vi "Demo.vi"() -> ()   [LabVIEW 2018]
doc: "Example API Tester."
uses:
  Classes/ExampleAPI/ExampleAPI.lvclass
panel:
  in  "Get Bitness Info":bool
  in  "machine name (\"\":  local reference)":string="localhost"
  in  "port number":u16=3365
  in  "wait for reply":bool=TRUE
  in  "X":dbl=1.0
  out "Reply Payload":dbl
  in  "Stop Module":bool
  in  "Test Do Something Else and Wait for Reply":bool
  in  "Hide Module Panel":bool
  in  "Show Module Panel":bool
  in  "Test Do Something Else":bool
  in  "Test Do Something":bool
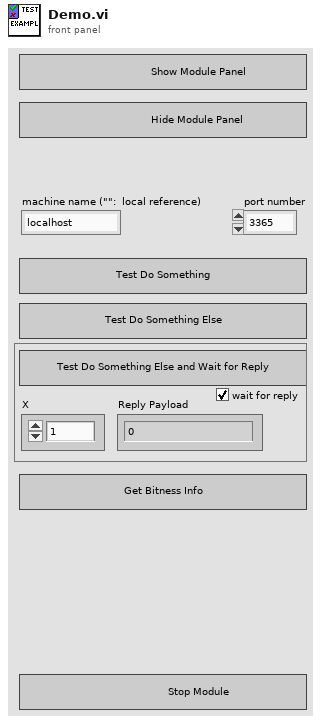
[diagram p1: front panel]
types:
  T1 = typedef "Example.lvlib/Do Something Else and Wait (Reply Payload)--cluster.ctl" = cluster{"Value":dbl, "error":errorcluster}
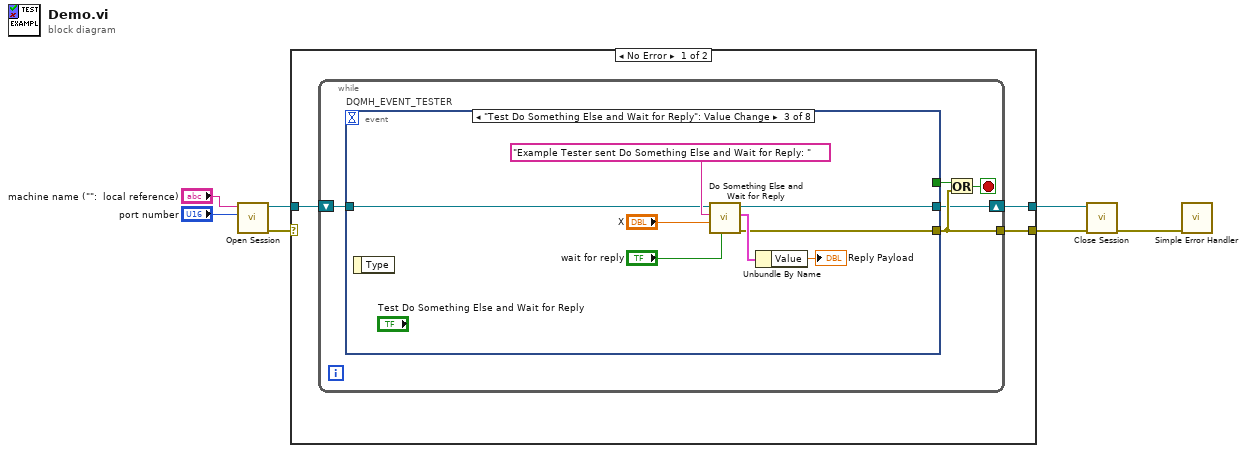
[diagram p0: block diagram]
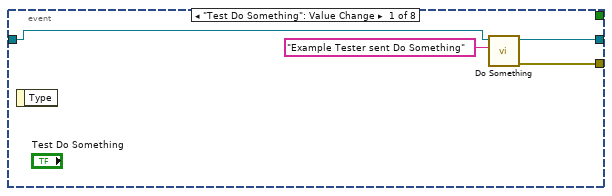
[diagram p2: hidden frame]
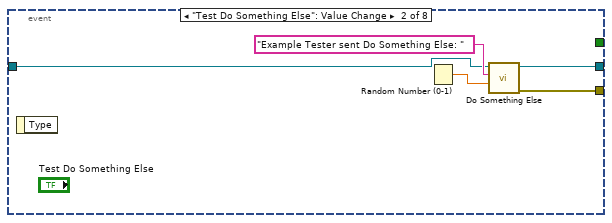
[diagram p3: hidden frame]
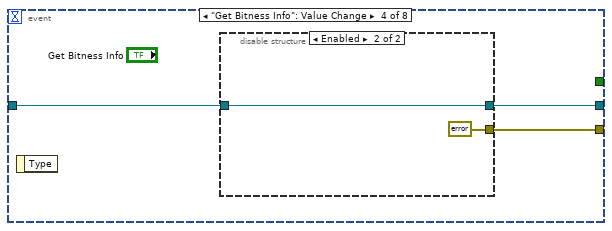
[diagram p4: hidden frame]
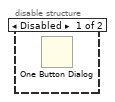
[diagram p5: hidden frame]
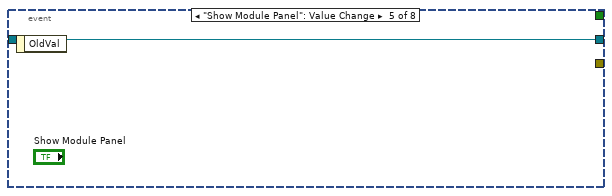
[diagram p6: hidden frame]
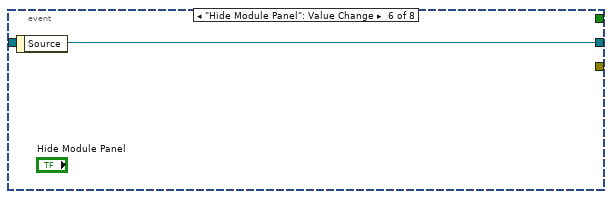
[diagram p7: hidden frame]
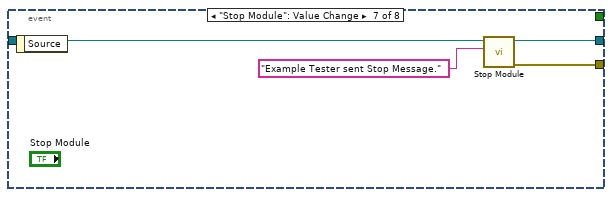
[diagram p8: hidden frame]
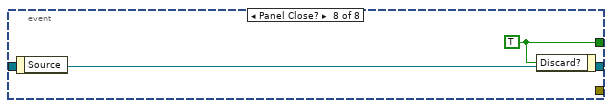
[diagram p9: hidden frame]
diagram:
  n1 = call "Open Session.vi"("port number or service name (3364)"="port number", "machine name (\"\":  local reference)"="machine name (\"\":  local reference)") -> ("error out"=w3:errorcluster, "ExampleAPI out"=w4:refnum<class "ExampleAPI.lvclass">)  [unwired: 8 in]
  n2 = case shown="No Error" w3 {
    selector: w3 -> [_ w47]
    tunnel: w4 -> [w10 w46]
    tunnel: [w9 w46] -> w7
    tunnel: [w8 w47] -> w6
    frame No Error {
      n3 = while {
        shift-right: [w11] -> w9
        shift-left: w10 -> [w12]
        tunnel: [w13] -> w8
        stop <- w14 stop-if-true
        n4 = event "DQMH_EVENT_TESTER" shown="[2] \"Test Do Something Else and Wait for Reply\": Value Change" {
          selector: _ -> [_ _ _ _ _ _ _ _]
          dyn-events: _ -> [_ _ _ _ _ _ _ _]
          timeout: _ -> [_ _ _ _ _ _ _ _]
          tunnel: [_ _ _ _ _ _ _ w45] -> w15
          tunnel: [w19 w24 w25 w33 _ _ w41 _] -> w13
          tunnel: w12 -> [w17 w21 w29 w35 w38 w39 w43 w44]
          tunnel: [w16 w20 w28 w34 w38 w39 w42 w44] -> w11
          event "Test Do Something": Value Change {
            n5 = event-data() -> ()  [unwired: 1 in, 1 out]
            n6 = call "Do Something.vi"("Do Something Message"="Example Tester sent Do Something", "TemplateAPI in"=w17) -> ("error out"=w19:errorcluster, "TemplateAPI out"=w16:refnum<class "ExampleAPI.lvclass">)  [unwired: 8 in]
          }
          event "Test Do Something Else": Value Change {
            n7 = event-data() -> ()  [unwired: 1 in, 1 out]
            n8 = Random Number (0-1)() -> (number: 0 to 1=w22:dbl)
            n9 = call "Do Something Else.vi"("X"=w22, "Do Something Message"="Example Tester sent Do Something Else: ", "TemplateAPI in"=w21) -> ("error out"=w24:errorcluster, "TemplateAPI out"=w20:refnum<class "ExampleAPI.lvclass">)  [unwired: 7 in]
          }
          event "Test Do Something Else and Wait for Reply": Value Change {
            n10 = event-data() -> ()  [unwired: 1 in, 1 out]
            n11 = call "Do Something Else and Wait for Reply.vi"("wait for reply (T)"="wait for reply", "X"="X", "Do Something Message"="Example Tester sent Do Something Else and Wait for Reply: ", "TemplateAPI in"=w29) -> ("error out"=w25:errorcluster, "Reply Payload"=w27:T1, "TemplateAPI out"=w28:refnum<class "ExampleAPI.lvclass">)  [unwired: 4 in, 1 out]
            n12 = Unbundle By Name(w27) -> ("Value"=→"Reply Payload":dbl)
          }
          event "Get Bitness Info": Value Change {
            n13 = event-data() -> ()  [unwired: 1 in, 1 out]
            n14 = disable-structure shown="Enabled" {
              disable-tunnel: w35 -> [_ w37]
              disable-tunnel: [_ w37] -> w34
              disable-tunnel: [_ errorcluster {"status"=FALSE, "code"=0, "source"=""} ("error constant")] -> w33
              frame Disabled {
                n15 = One Button Dialog() -> ()  [unwired: 2 in, 1 out]
              }
              frame Enabled {
              }
            }
          }
          event "Show Module Panel": Value Change {
            n16 = event-data() -> ()  [unwired: 1 in, 1 out]
          }
          event "Hide Module Panel": Value Change {
            n17 = event-data() -> ()  [unwired: 1 in, 1 out]
          }
          event "Stop Module": Value Change {
            n18 = event-data() -> ()  [unwired: 1 in, 1 out]
            n19 = call "Stop Module.vi"("Origin"="Example Tester sent Stop Message.", "TemplateAPI in"=w43) -> ("error out"=w41:errorcluster, "TemplateAPI out"=w42:refnum<class "ExampleAPI.lvclass">)  [unwired: 8 in]
          }
          event Panel Close? {
            w45 = TRUE ("Discard?")
            n20 = event-data() -> ()  [unwired: 1 in, 1 out]
            n21 = event-data("Discard?"=w45) -> ()  [unwired: 1 in, 1 out]
          }
        }
        n22 = Or(x=w15, y=w13) -> (x .or. y?=w14:bool)
      }
    }
    frame Error {
    }
  }
  n23 = call "Close Session.vi"("error in (no error)"=w6, "ExampleAPI.lvclass"=w7) -> ("error out"=w5:errorcluster)  [unwired: 9 in]
  n24 = call <vilib>:"Simple Error Handler.vi"("error in (no error)"=w5) -> ()  [unwired: 4 in, 5 out]
